vi "Packet Read Header.vi"(8 "error in (no error)":errorcluster, 10 "Data":u8[](array[numeric]), 11 "Map in":refnum<class "Map.lvclass">) -> (0 "error out":errorcluster, 3 "Map out":refnum<class "Map.lvclass">)   [LabVIEW 2019, in "Map.lvclass"]
uses:
  Map.lvclass
  TCP Packet/Packet.lvclass
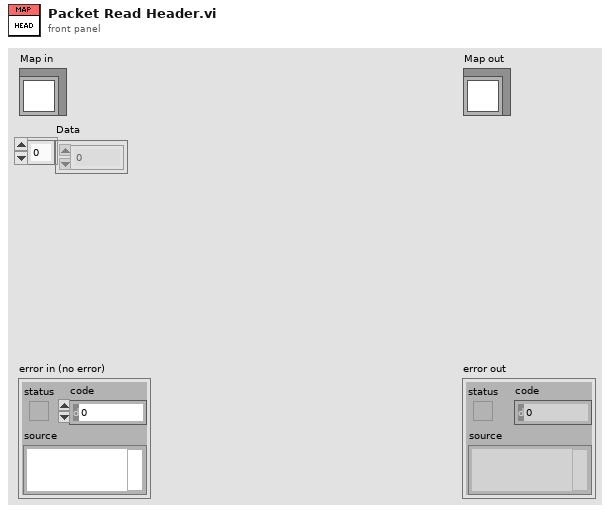
[diagram p1: front panel]
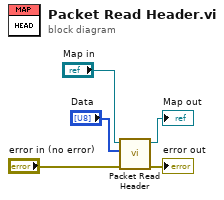
[diagram p0: block diagram]
diagram:
  n1 = call-parent "Packet Read Header.vi"("error in (no error)"="error in (no error)", "Data"="Data", "Packet in"="Map in") -> ("error out"=→"error out":errorcluster, "Packet out"=→"Map out":refnum<class "Map.lvclass">)  [unwired: 7 in]
